vi "Parse design request.vi"(11 "Request":T3={"Key"=["SERVER_PROTOCOL", "SERVER_SOFTWARE", "GATEWAY_INTERFACE", "SERVER_PORT", "SERVER_NAME", "DOCUMENT_ROOT", "SERVER_URL", "SERVER_ADDR", "SERVER_HOST", "QUERY_STRING", "CONTENT_LENGTH", "PATH_INFO", "SCRIPT_FILENAME", "AUTH_TYPE", "REMOTE_HOST", "SERVICE_NAME", "REQUEST_URI", "SERVICE_PATH", "REQUEST_TRANSPORT", "SCRIPT_NAME", "CONTENT_TYPE", "PATH_TRANSLATED", "REMOTE_USER", "REMOTE_ADDR", "REQUEST_METHOD", "CONTENT_LENGTH", "HOST", "CONNECTION", "REFERER", "ACCEPT", "COOKIE", "CACHE_CONTROL", "ACCEPT_ENCODING", "CONTENT_TYPE", "ACCEPT_CHARSET", "ACCEPT_LANGUAGE", "USER_AGENT", "ORIGIN", "HTTP_COOKIE", "ProjectCity", "Language", "Country", "ProjectTitle", "Email", "Name", "Organization", "Q.Plant[L/s]", "ProjectNotes", "ProjectState"], "Value"=["HTTP/1.1", "Mbedthis-Appweb/2.5.0", "CGI/1.1", "8080", "NI Application Web Server", "c:/program files/national instruments/shared/ni webserver/www", "NI Application Web Server", "", "NI Application Web Server", "", "227", "", "c:/program files/national instruments/shared/ni webserver/www/adt/adt", "", "132.236.94.39", "adt", "/ADT/ADT", "C:\\ProgramData\\National Instruments\\WebServices\\aws\\ADT-1CDAB8E2-A8D3-4514-B8CE-FE2D2119849A\\", "http", "/adt/adt", "application/x-www-form-urlencoded", "", "", "132.236.94.39", "POST", "227", "designserver.cee.cornell.edu:8080", "keep-alive", "http://designserver.cee.cornell.edu:8080/adt/data/EtFlocSedFi.html", "text/html,application/xhtml+xml,application/xml;q=0.9,*/*;q=0.8", "__qca=P0-443584428-1305594823145; __utma=67039164.2078665383.1313933611.1329475713.1329843203.19; __utmz=67039164.1313933611.1.1.utmcsr=(direct)|utmccn=(direct)|utmcmd=(none); __utma=23486248.2063678279.1321994688.1329853680.1330380653.23; __utmz=23486248.1329853680.22.5.utmcsr=google|utmccn=(organic)|utmcmd=organic|utmctr=(not%20provided); __unam=eda27ea-13048aaac3b-7928d9ad-479; BALANCEID=balancer.cf094; cuwltgttime=\"1331246035\"", "max-age=0", "gzip,deflate,sdch", "application/x-www-form-urlencoded", "ISO-8859-1,utf-8;q=0.7,*;q=0.3", "en-US,en;q=0.8,es;q=0.6", "Mozilla/5.0 (Windows NT 6.1; WOW64) AppleWebKit/535.11 (KHTML, like Gecko) Chrome/17.0.963.56 Safari/535.11", "http://designserver.cee.cornell.edu:8080", "__qca=P0-443584428-1305594823145; __utma=67039164.2078665383.1313933611.1329475713.1329843203.19; __utmz=67039164.1313933611.1.1.utmcsr=(direct)|utmccn=(direct)|utmcmd=(none); __utma=23486248.2063678279.1321994688.1329853680.1330380653.23; __utmz=23486248.1329853680.22.5.utmcsr=google|utmccn=(organic)|utmcmd=organic|utmctr=(not%20provided); __unam=eda27ea-13048aaac3b-7928d9ad-479; BALANCEID=balancer.cf094; cuwltgttime=\"1331246035\"", "Ithaca", "English", "US", "testing agian", "mw24@cornell.edu", "Cornell University", "Cornell University", "2145", "lots of water", "New York"]}) -> (0 "Good Method":bool, 1 "Design inputs":T1, 2 "User and project info":T1, 3 "Method":string)   [LabVIEW 2012, in "Design Server.lvlib"]
uses:
  Design Server.lvlib
  Variable cluster.ctl
  user project design.ctl
  RequestKeys.ctl
panel:
  in  "datatype":T1
  in  "Request Keys":T2=enum."ProjectNotes"
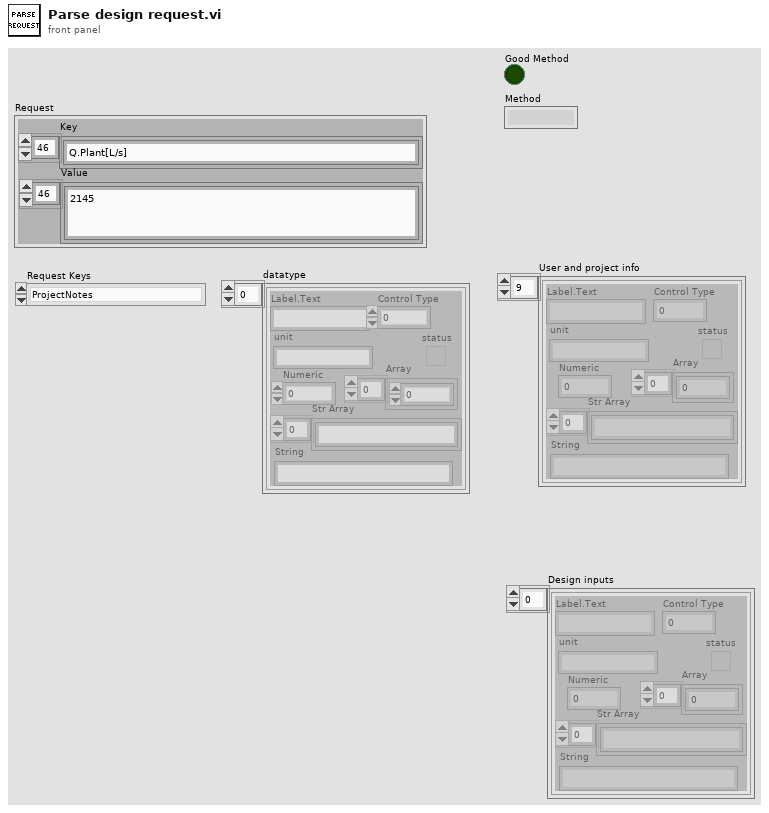
[diagram p1: front panel]
types:
  T1 = typedef "Design Server.lvlib/Variable cluster.ctl" = cluster{"Label.Text":string, "Control Type":u32, "Numeric":dbl, "Array":dbl[], "status":bool, "Str Array":string[], "String":string, "unit":string}[]
  T2 = typedef "Design Server.lvlib/RequestKeys.ctl" = enum16{"FormName", "Name", "Email", "Organization", "Country", "ProjectTitle", "ProjectCity", "ProjectState", "ProjectNotes"}
  T3 = typedef "Design Server.lvlib/user project design.ctl" = cluster{"Key":string[], "Value":string[]}
  T4 = cluster{"Label.Text":string, "Control Type":u32, "Numeric":dbl, "Array":dbl[], "status":bool, "Str Array":string[], "String":string, "unit":string}
  T5 = cluster{"Label.Text":string, "Control Type":u32, "Numeric":dbl, "Array":dbl[], "status":bool, "Str Array":string[], "String":string, "unit":string}[]
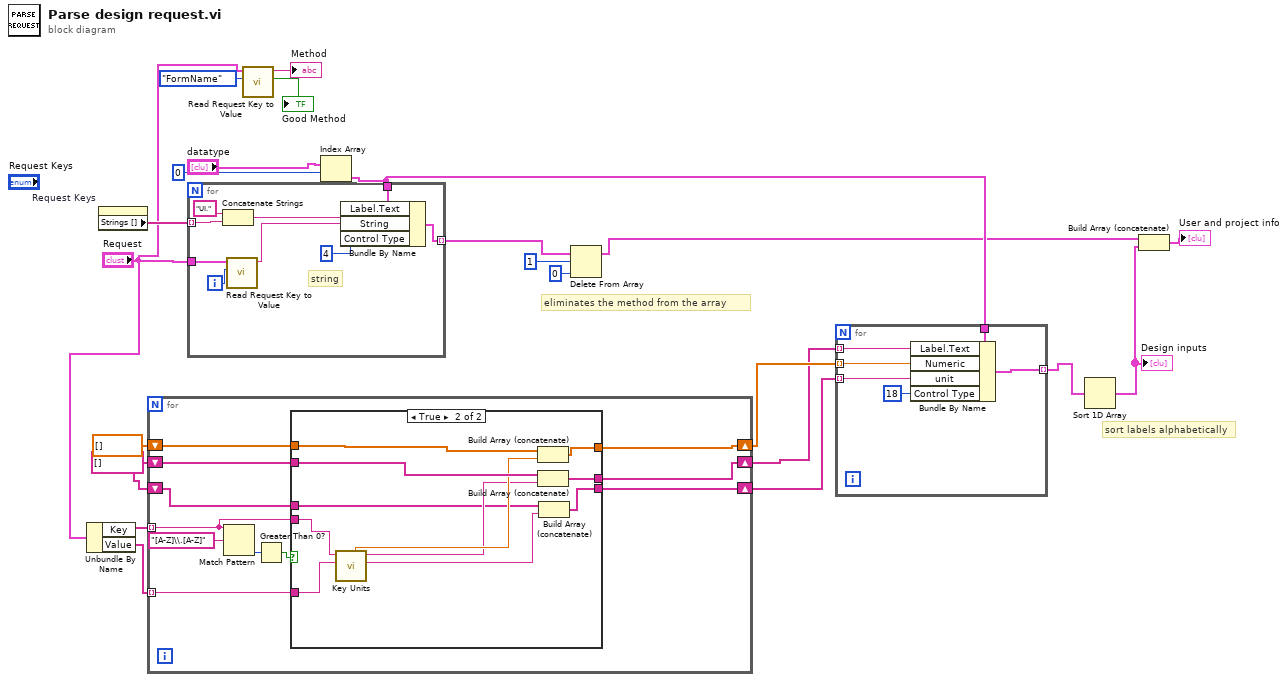
[diagram p0: block diagram]
diagram:
  w5 = string[] []
  # "sort labels alphabetically"
  # "eliminates the method from the array"
  n1 = Unbundle By Name("Request") -> ("Key"=w19:string[], "Value"=w18:string[])
  n2 = property on="Request Keys" class="Enum (strict)"() -> ("Strings []"=w22:string[])  [unwired: 2 in, 2 out]
  n3 = for {
    tunnel: w19 -> [w25] mode=indexing
    shift-right: [w30] -> w15
    shift-left: dbl[] [] -> [w29]
    tunnel: w18 -> [w31] mode=indexing
    shift-right: [w27] -> w14
    shift-left: w5 -> [w28]
    shift-right: [w24] -> w6
    shift-left: w5 -> [w23]
    n4 = Match Pattern(string=w25, regular expression="[A-Z]\\.[A-Z]") -> (offset past match=w32:i32)  [unwired: 1 in, 3 out]
    n5 = Greater Than 0?(x=w32) -> (x > 0?=w26:bool)
    n6 = case shown="True" w26 {
      tunnel: w31 -> [_ w44]
      tunnel: [w36 w47] -> w30
      tunnel: w29 -> [w36 w46]
      tunnel: w28 -> [w35 w45]
      tunnel: [w35 w40] -> w27
      tunnel: w25 -> [_ w43]
      tunnel: [w34 w38] -> w24
      tunnel: w23 -> [w34 w37]
      frame False {
      }
      frame True {
        n7 = call "Key Units.vi"("Value"=w44, "Key"=w43) -> ("Units"=w39:string, "Variable Name"=w41:string, "number"=w42:dbl)  [unwired: 7 in]
        n8 = Build Array (concatenate)(w46, w42) -> (w47:dbl[])
        n9 = Build Array (concatenate)(w45, w41) -> (w40:string[])
        n10 = Build Array (concatenate)(w37, w39) -> (w38:string[])
      }
    }
  }
  n11 = call "Read Request Key to Value.vi"("Request Keys"=RequestKeys."FormName", "Request"="Request") -> ("Found Key"=→"Good Method":bool, "Value"=→"Method":string)  [unwired: 8 in]
  n12 = Index Array(array="datatype", index=0) -> (element=w16:T4)
  n13 = for {
    tunnel: "Request" -> [w56]
    tunnel: w22 -> [w54] mode=indexing
    tunnel: [w53] -> w9 mode=indexing
    tunnel: w16 -> [w50]
    i -> [w55]
    # "string"
    n14 = Concatenate Strings("UI." ("string"), w54) -> (w52:string)
    n15 = call "Read Request Key to Value.vi"("Request Keys"=w55, "Request"=w56) -> ("Value"=w49:string)  [unwired: 8 in, 1 out]
    n16 = Bundle By Name(cluster=w50, "Label.Text"=w52, "String"=w49, "Control Type"=u32 4) -> (w53:T4)
  }
  n17 = Delete From Array(array=w9, length=1, index=0) -> (array with subset deleted=w8:T5)  [unwired: 1 out]
  n18 = for {
    tunnel: w16 -> [w62]
    tunnel: w15 -> [w61] mode=indexing
    tunnel: w14 -> [w60] mode=indexing
    tunnel: [w59] -> w2 mode=indexing
    tunnel: w6 -> [w57] mode=indexing
    n19 = Bundle By Name(cluster=w62, "Label.Text"=w60, "Numeric"=w61, "unit"=w57, "Control Type"=u32 18) -> (w59:T4)
  }
  n20 = Sort 1D Array(array=w2) -> (sorted array=w1:T5)
  "Design inputs" <- w1
  n21 = Build Array (concatenate)(w8, w1) -> (→"User and project info":T5)
